vi "Write Data.vi"(8 "error in (no error)":errorcluster, 9 "Publication Time":timestamp, 10 "Value":variant, 11 "ActorMessageTransport In":refnum<class "ActorMessageTransport.lvclass">) -> (0 "error out":errorcluster, 3 "ActorMessageTransport Out":refnum<class "ActorMessageTransport.lvclass">)   [LabVIEW 2020, in "ActorMessageTransport.lvlib" / "ActorMessageTransport.lvclass"]
doc: "写入数据"
uses:
  ActorMessageTransport.lvclass
  ActorMessageTransport.lvclass/ActorMessageTransport.ctl
  <vilib>/Utility/error.llb/Error Cluster From Error Code.vi
  <vilib>/ErrorRing/Error Ring.xnode
  Notification Msg/Notification Msg.lvclass
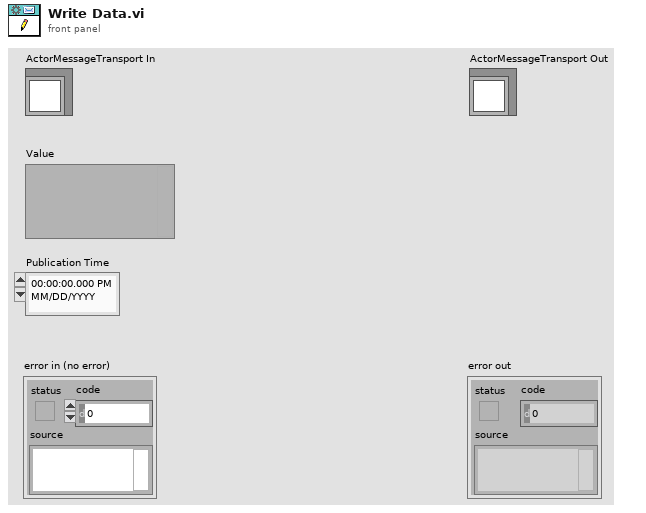
[diagram p1: front panel]
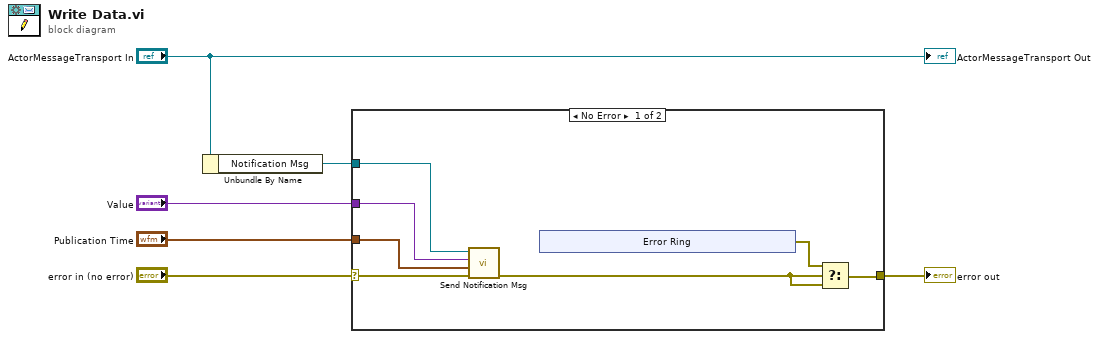
[diagram p0: block diagram]
diagram:
  n1 = Unbundle By Name("ActorMessageTransport In") -> ("Notification Msg"=w6:refnum<class "Notification Msg.lvclass">)
  n2 = case shown="No Error" "error in (no error)" {
    selector: "error in (no error)" -> [w10 w19]
    tunnel: w6 -> [w13 _]
    tunnel: "Value" -> [w12 _]
    tunnel: "Publication Time" -> [w11 _]
    tunnel: [w9 w19] -> w1
    frame No Error {
      n3 = call-dynamic "Send Notification Msg.vi"("error in (no error)"=w10, "Publication Time (Use Current Time)"=w11, "Value"=w12, "Notification Msg"=w13) -> ("error out"=w8:errorcluster)  [unwired: 7 in]
      n4 = xnode "Error Ring"() -> ("error out"=w7:errorcluster)
      n5 = Select(t=w7, s=w8, f=w8) -> (s? t:f=w9:errorcluster)
    }
    frame Error {
    }
  }
  "error out" <- w1
  "ActorMessageTransport Out" <- "ActorMessageTransport In"
